vi "VIS-IR_FFRS.vi"(8 "error in (no error)":errorcluster, 11 "VIS-IR in":refnum<class "VIS-NIR.lvclass">) -> (0 "error out":errorcluster, 3 "VIS-IR out":refnum<class "VIS-NIR.lvclass">)   [LabVIEW 2015, in "VIS-NIR.lvclass"]
uses:
  VIS-NIR.lvclass
  Detector.lvclass/Detector.ctl
  Detector.lvclass
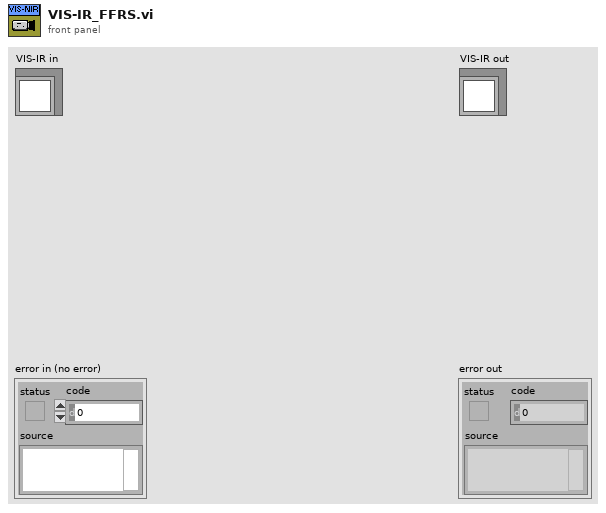
[diagram p1: front panel]
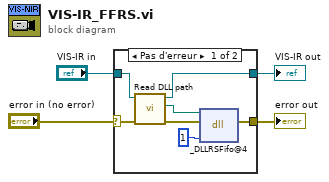
[diagram p0: block diagram]
diagram:
  n1 = case shown="Pas d'erreur" "error in (no error)" {
    selector: "error in (no error)" -> [w10 w13]
    tunnel: [w7 w13] -> w3
    tunnel: [w5 w12] -> w1
    tunnel: "VIS-IR in" -> [w11 w12]
    frame No Error {
      n2 = call "Read DLL path.vi"("error in (no error)"=w10, "Detector in"=w11) -> ("error out"=w9:errorcluster, "DLL path"=w6:path, "Detector out"=w5:refnum<class "VIS-NIR.lvclass">)  [unwired: 7 in]
      n3 = dll-call lib="G:/SD/TRANCON/DLL/ESLSCDLL.dll" fn="_DLLRSFifo@4" ("lwlscdll.dll:DLLRSFifo")(path in=w6, error in=w9, "drv"=u32 1) -> (error out=w7:errorcluster)  [unwired: 3 in, 1 out]
    }
    frame Error {
    }
  }
  "error out" <- w3
  "VIS-IR out" <- w1
